vi "Read.vi"(8 "error in":errorcluster, 11 "PCAN in":refnum<class "PCAN.lvclass">) -> (0 "error out":errorcluster, 2 "CAN Message":T1 {"MSG type" format="%x"; "ID" format="%.0x"}, 3 "PCAN out":refnum<class "PCAN.lvclass">)   [LabVIEW 2024, in "PCAN.lvclass"]
uses:
  PCAN.lvclass
  PCAN.lvclass/PCAN.ctl
  Configurations/CFG Base/CFG Base.lvclass
  D:/git/HAL/HAL/Configurations/CFG Base/CFG Base.lvclass
  D:/git/HAL/HAL/Devices/CAN Interfaces/PCAN/PCAN.lvclass
  D:/git/HAL/HAL/Protocols/ICAN/ICAN.lvclass
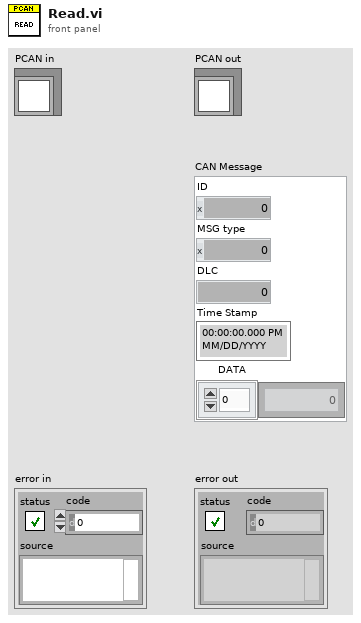
[diagram p1: front panel]
types:
  T1 = cluster{"ID":u32, "MSG type":u8, "DLC":u8, "Time Stamp":timestamp, "DATA":u8[]}
  T2 = typedef "TPCANHandle.ctl" = enum16{"PCAN_NONEBUS  0x000", "PCAN_ISABUS1  0x21", "PCAN_ISABUS2  0x22", "PCAN_ISABUS3  0x23", "PCAN_ISABUS4  0x24", "PCAN_ISABUS5  0x25", "PCAN_ISABUS6  0x26", "PCAN_ISABUS7  0x27", "PCAN_ISABUS8  0x28", "PCAN_DNGBUS1  0x31", "PCAN_PCIBUS1  0x41", "PCAN_PCIBUS1  0x42", "PCAN_PCIBUS1  0x43", "PCAN_PCIBUS1  0x44", "PCAN_PCIBUS1  0x45", "PCAN_PCIBUS1  0x46", "PCAN_PCIBUS1  0x47", "PCAN_PCIBUS1  0x48", "PCAN_PCIBUS1  0x409", "PCAN_PCIBUS1  0x40A", "PCAN_PCIBUS1  0x40B", "PCAN_PCIBUS1  0x40C", "PCAN_PCIBUS1  0x40D", "PCAN_PCIBUS1  0x40E", "PCAN_PCIBUS1  0x40F", "PCAN_PCIBUS1  0x410", "PCAN_USBBUS1  0x51", "PCAN_USBBUS2  0x52", "PCAN_USBBUS3  0x53", "PCAN_USBBUS4  0x54", "PCAN_USBBUS5  0x55", "PCAN_USBBUS6  0x56", "PCAN_USBBUS7  0x57", "PCAN_USBBUS8  0x58", "PCAN_USBBUS9  0x509", "PCAN_USBBUS10  0x50A", "PCAN_USBBUS11  0x50B", "PCAN_USBBUS12  0x50C", "PCAN_USBBUS13  0x50D", "PCAN_USBBUS14  0x50E", "PCAN_USBBUS15  0x50F", "PCAN_USBBUS16  0x510", "PCAN_PCCBUS1  0x61", "PCAN_PCCBUS2  0x62", "PCAN_LANBUS1  0x801", "PCAN_LANBUS2  0x802", "PCAN_LANBUS3  0x803", "PCAN_LANBUS4  0x804", "PCAN_LANBUS5  0x805", "PCAN_LANBUS6  0x806", "PCAN_LANBUS7  0x807", "PCAN_LANBUS8  0x808", "PCAN_LANBUS9  0x809", "PCAN_LANBUS10  0x80A", "PCAN_LANBUS11  0x80B", "PCAN_LANBUS12  0x80C", "PCAN_LANBUS13  0x80D", "PCAN_LANBUS14  0x80E", "PCAN_LANBUS15  0x80F", "PCAN_LANBUS16  0x810"}
  T3 = typedef "TPCANTimestamp.ctl" = cluster{"millis overflow":u16, "millis ":u32, "micros":u16}
  T4 = typedef "CAN MSG Cluster.ctl" = cluster{"ID":u32, "MSG type":u8, "DLC":u8, "DATA":u8[]}
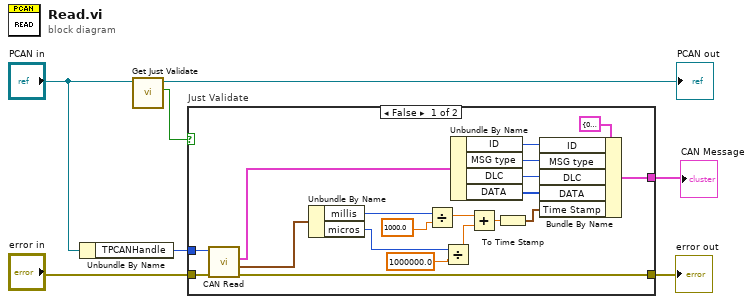
[diagram p0: block diagram]
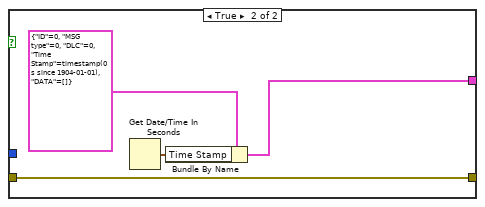
[diagram p2: hidden frame]
diagram:
  n1 = Unbundle By Name("PCAN in") -> ("TPCANHandle"=w6:T2)
  n2 = call "Get Just Validate.vi"("CFG Base in"="PCAN in") -> ("Just Validate"=w4:bool, "CFG Base out"=→"PCAN out":refnum<class "PCAN.lvclass">)  [unwired: 9 in]
  n3 = case "Just Validate" shown="False" w4 {
    tunnel: w6 -> [w26 _]
    tunnel: "error in" -> [w25 w30]
    tunnel: [w24 w30] -> w2
    tunnel: [w8 w27] -> w1
    frame False {
      n4 = call <instrlib>:"CAN Read.vi"("error in (no error)"=w25, "TPCANHandle"=w26) -> ("error out"=w24:errorcluster, "TPCANTimestamp out"=w15:T3, "CAN_Message out"=w14:T4)  [unwired: 5 in, 2 out]
      n5 = Unbundle By Name(w15) -> ("millis"=w23:u32, "micros"=w21:u16)
      n6 = Divide(x=w23, y=1000.0) -> (x/y=w17:dbl)
      n7 = Divide(x=w21, y=1000000.0) -> (x/y=w18:dbl)
      n8 = Unbundle By Name(w14) -> ("ID"=w13:u32, "MSG type"=w9:u8, "DLC"=w10:u8, "DATA"=w11:u8[])
      n9 = Add(x=w17, y=w18) -> (x+y=w19:dbl)
      n10 = To Time Stamp(1:w19) -> (0:w12:timestamp)
      n11 = Bundle By Name(cluster=T1 {"ID"=0, "MSG type"=0, "DLC"=0, "Time Stamp"=timestamp(0 s since 1904-01-01), "DATA"=[]} ("CAN Message"), "ID"=w13, "MSG type"=w9, "DLC"=w10, "DATA"=w11, "Time Stamp"=w12) -> (w8:T1)
    }
    frame True {
      n12 = Get Date/Time In Seconds() -> (seconds since 1Jan1904=w28:timestamp)
      n13 = Bundle By Name(cluster=T1 {"ID"=0, "MSG type"=0, "DLC"=0, "Time Stamp"=timestamp(0 s since 1904-01-01), "DATA"=[]} ("CAN Message"), "Time Stamp"=w28) -> (w27:T1)
    }
  }
  "error out" <- w2
  "CAN Message" <- w1
